vi "XLP80_Action_Scroll.vi"(8 "err in":errorcluster, 11 "Refs":T1) -> (0 "err out":errorcluster)   [LabVIEW 2021]
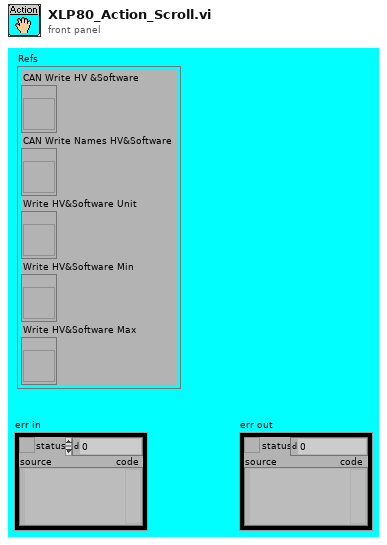
[diagram p1: front panel]
types:
  T1 = cluster{"CAN Write HV &Software":refnum<vi>, "CAN Write Names HV&Software":refnum<vi>, "Write HV&Software Unit":refnum<vi>, "Write HV&Software Min":refnum<vi>, "Write HV&Software Max":refnum<vi>}
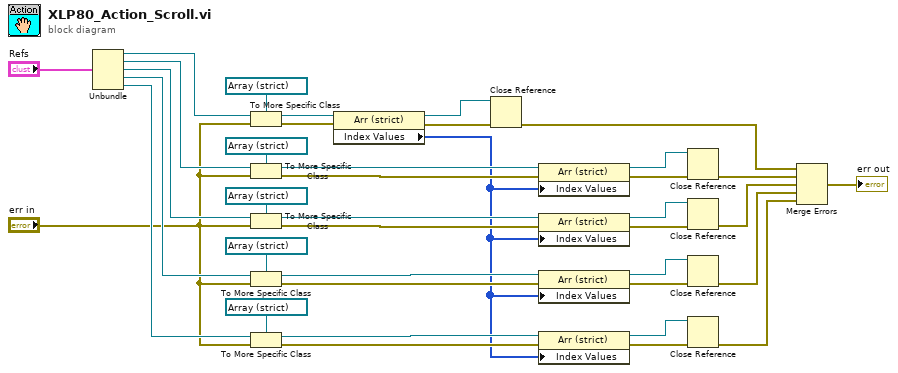
[diagram p0: block diagram]
diagram:
  n1 = Unbundle("Refs") -> ("CAN Write HV &Software"=w26:refnum<vi>, "CAN Write Names HV&Software"=w25:refnum<vi>, "Write HV&Software Unit"=w19:refnum<vi>, "Write HV&Software Min"=w17:refnum<vi>, "Write HV&Software Max"=w7:refnum<vi>)
  n2 = To More Specific Class(target class=refnum<vi> refnum ("FB CAN Write"), reference=w26, error in="err in") -> (specific class reference=w36:refnum<vi>, error out=w37:errorcluster)
  n3 = To More Specific Class(target class=refnum<vi> refnum ("CAN Write Names"), reference=w25, error in="err in") -> (specific class reference=w35:refnum<vi>, error out=w34:errorcluster)
  n4 = To More Specific Class(target class=refnum<vi> refnum ("CAN Write Names"), reference=w19, error in="err in") -> (specific class reference=w21:refnum<vi>, error out=w22:errorcluster)
  n5 = To More Specific Class(target class=refnum<vi> refnum ("FB CAN Write"), reference=w17, error in="err in") -> (specific class reference=w14:refnum<vi>, error out=w13:errorcluster)
  n6 = To More Specific Class(target class=refnum<vi> refnum ("FB CAN Write"), reference=w7, error in="err in") -> (specific class reference=w11:refnum<vi>, error out=w12:errorcluster)
  n7 = property class="Arr (strict)"(reference=w36, error in=w37) -> (reference out=w32:refnum<vi>, error out=w33:errorcluster, "Index Values"=w5:u32[])
  n8 = Close Reference(reference=w32, error in (no error)=w33) -> (error out=w28:errorcluster)
  n9 = property class="Arr (strict)"(reference=w35, error in=w34, "Index Values"=w5) -> (reference out=w30:refnum<vi>, error out=w31:errorcluster)
  n10 = property class="Arr (strict)"(reference=w21, error in=w22, "Index Values"=w5) -> (reference out=w24:refnum<vi>, error out=w23:errorcluster)
  n11 = property class="Arr (strict)"(reference=w14, error in=w13, "Index Values"=w5) -> (reference out=w15:refnum<vi>, error out=w16:errorcluster)
  n12 = property class="Arr (strict)"(reference=w11, error in=w12, "Index Values"=w5) -> (reference out=w10:refnum<vi>, error out=w9:errorcluster)
  n13 = Close Reference(reference=w30, error in (no error)=w31) -> (error out=w29:errorcluster)
  n14 = Close Reference(reference=w24, error in (no error)=w23) -> (error out=w4:errorcluster)
  n15 = Close Reference(reference=w15, error in (no error)=w16) -> (error out=w3:errorcluster)
  n16 = Close Reference(reference=w10, error in (no error)=w9) -> (error out=w2:errorcluster)
  n17 = Merge Errors(w28, w29, w4, w3, w2) -> (→"err out":errorcluster)
